vi "Init State.vi"() -> (3 "Main State":T1)   [LabVIEW 2019, in "UI.lvlib"]
uses:
  UI.lvlib
  Main States.ctl
  UI Message Queue.ctl
  Update Message.ctl
  Update Command.ctl
  Controller/Controller Message Queue.ctl
  Controller/Controller Message.ctl
  Controller/MDS Command.ctl
  Listener/Listener Message Queue.ctl
  Listener/Listener Message.ctl
  Listener/Listener Command.ctl
  Controller/Controller.lvlib
  Listener/Listener.lvlib
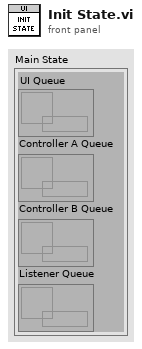
[diagram p1: front panel]
types:
  T1 = typedef "UI.lvlib/Main States.ctl" = cluster{"UI Queue":T2, "Controller A Queue":T3, "Controller B Queue":T3, "Listener Queue":T4}
  T2 = typedef "UI.lvlib/UI Message Queue.ctl" = refnum<queue>
  T3 = typedef "Controller.lvlib/Controller Message Queue.ctl" = refnum<queue>
  T4 = typedef "Listener.lvlib/Listener Message Queue.ctl" = refnum<queue>
  T5 = typedef "Listener.lvlib/Listener Message.ctl" = cluster{"Listener Command":T6, "Value":variant}
  T6 = typedef "Listener.lvlib/Listener Command.ctl" = enum16{"Idle", "Open", "Incoming", "Close", "Error", "Stop"}
  T7 = typedef "Controller.lvlib/Controller Message.ctl" = cluster{"MDS Command":T8, "Channel":u8, "Value":variant}
  T8 = typedef "Controller.lvlib/MDS Command.ctl" = enum16{"Idle", "Open", "Set VMode", "Set IMode", "Get Frequency", "Set Frequency", "Get Power", "Set Power (dBm)", "Set Power (%)", "Get Switch", "Switch Channel", "Store", "Wait for Prompt", "Wait for State", "Reset", "Error", "Close", "Stop"}
  T9 = typedef "UI.lvlib/Update Message.ctl" = cluster{"Update Command":T10, "Channel":u8, "Value":variant}
  T10 = typedef "UI.lvlib/Update Command.ctl" = enum16{"Update Frequency", "Update Power", "Update Switch", "Error", "Stop"}
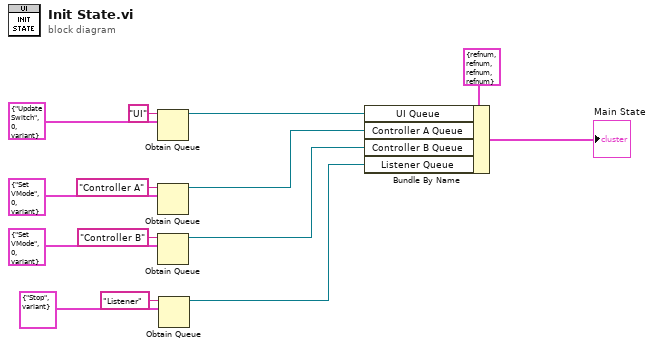
[diagram p0: block diagram]
diagram:
  n1 = Obtain Queue(name (unnamed)="UI", element data type=T9 {"Update Command"=enum."Update Switch", "Channel"=0, "Value"=variant} ("Controller Message")) -> (queue out=w13:refnum<queue>)  [unwired: 3 in, 2 out]
  n2 = Obtain Queue(name (unnamed)="Controller A", element data type=T7 {"MDS Command"=enum."Set VMode", "Channel"=0, "Value"=variant} ("Controller Message")) -> (queue out=w9:refnum<queue>)  [unwired: 3 in, 2 out]
  n3 = Obtain Queue(name (unnamed)="Controller B", element data type=T7 {"MDS Command"=enum."Set VMode", "Channel"=0, "Value"=variant} ("Controller Message")) -> (queue out=w7:refnum<queue>)  [unwired: 3 in, 2 out]
  n4 = Obtain Queue(name (unnamed)="Listener", element data type=T5 {"Listener Command"=enum."Stop", "Value"=variant} ("Listener Message")) -> (queue out=w1:refnum<queue>)  [unwired: 3 in, 2 out]
  n5 = Bundle By Name(cluster=T1 {"UI Queue"=refnum, "Controller A Queue"=refnum, "Controller B Queue"=refnum, "Listener Queue"=refnum} ("States"), "UI Queue"=w13, "Controller A Queue"=w9, "Controller B Queue"=w7, "Listener Queue"=w1) -> (→"Main State":T1)
